vi "Write Valve.vi"(8 "error in (no error)":errorcluster, 11 "MFC in":refnum<class "Valve.lvclass">) -> (0 "error out":errorcluster, 3 "MFC out":refnum<class "Valve.lvclass">)   [LabVIEW 2013, in "Valve.lvlib" / "Valve.lvclass"]
uses:
  Valve.lvclass
  Valve.lvclass/Valve.ctl
  Read Valve Position.vi
  Read VISA.vi
  PluginInterface/PluginInterface.lvlibp/PluginInterfaceClass/Read DVR.vi
  PluginInterface/Actor Framework.lvlibp/Message Enqueuer/Enqueue.vi
  Valve Messages/Log Data Msg/Log Data Msg.lvclass
  Valve Messages/Update Graphs Msg/Update Graphs Msg.lvclass
  PluginInterface/Actor Framework.lvlibp/Actor/Actor.lvclass
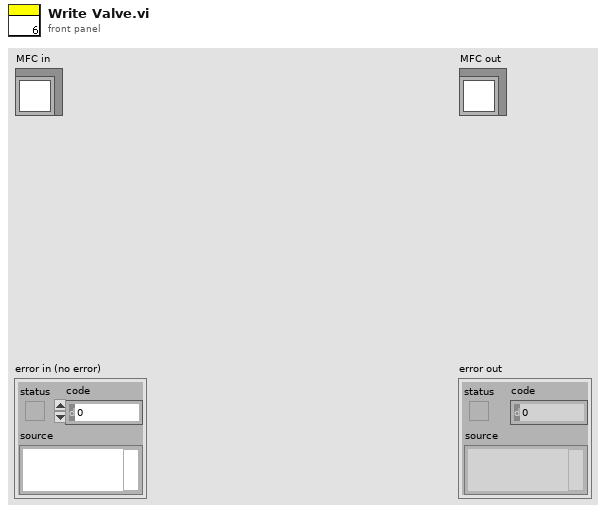
[diagram p1: front panel]
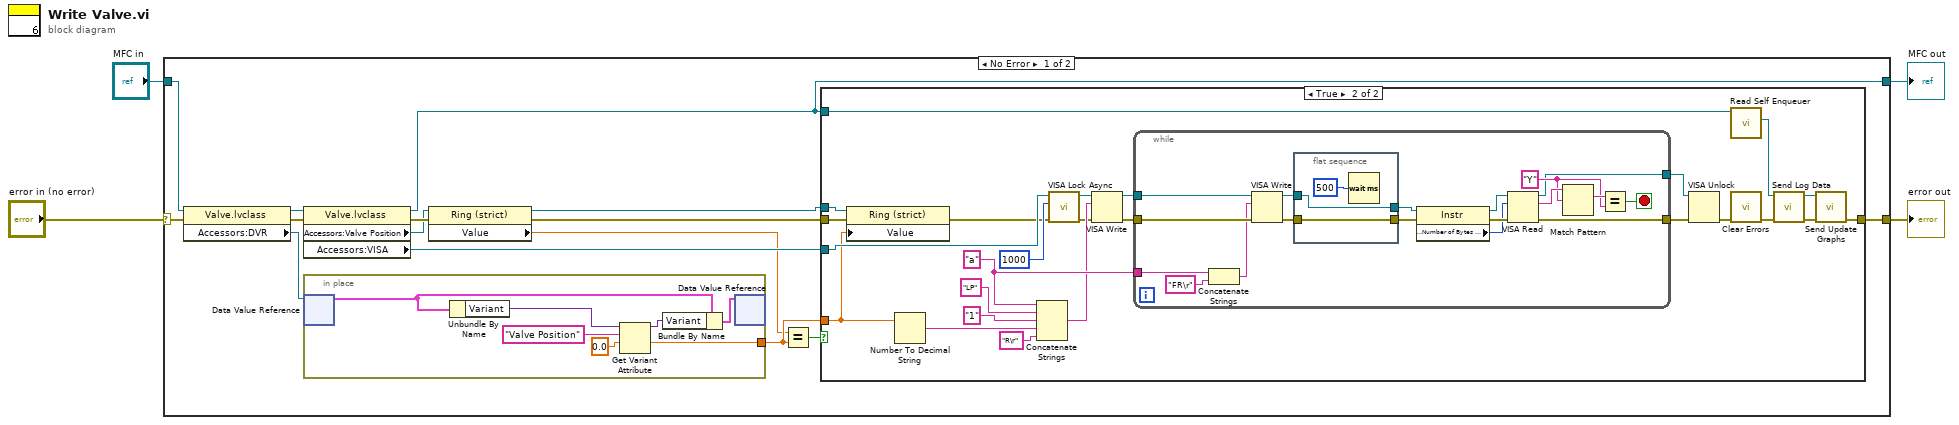
[diagram p0: block diagram]
diagram:
  n1 = case shown="No Error" "error in (no error)" {
    selector: "error in (no error)" -> [w18 w75]
    tunnel: [w12 w75] -> w1
    tunnel: [w5 w74] -> w2
    tunnel: "MFC in" -> [w19 w74]
    frame No Error {
      n2 = property class="Valve.lvclass"(reference=w19, error in=w18) -> (reference out=w17:refnum<class "Valve.lvclass">, error out=w15:errorcluster, "Accessors:DVR"=w16:refnum<data-value>)
      n3 = property class="Valve.lvclass"(reference=w17, error in=w15) -> (reference out=w5:refnum<class "Valve.lvclass">, error out=w14:errorcluster, "Accessors:Valve Position"=w13:refnum<vi>, "Accessors:VISA"=w11:refnum<visa-resource-name>)
      n4 = in-place {
        in-place-border: [w67] -> w7
        n5 = in-place-dvr #1(w16) -> (w70:cluster{"Array":string[], "Variant":variant})  [unwired: 1 out]
        n6 = Unbundle By Name(w70) -> ("Variant"=w72:variant)
        n7 = Get Variant Attribute(Variant=w72, name="Valve Position", default value (empty Variant)=0.0) -> (duplicate Variant=w71:variant, value=w67:dbl)  [unwired: 1 in, 2 out]
        n8 = Bundle By Name(cluster=w70, "Variant"=w71) -> (w73:cluster{"Array":string[], "Variant":variant})
        n9 = in-place-dvr #1(w73) -> ()  [unwired: 2 out]
      }
      n10 = property class="Ring (strict)"(reference=w13, error in=w14) -> (reference out=w10:refnum<vi>, error out=w9:errorcluster, "Value"=w6:dbl)
      n11 = Equal?(x=w6, y=w7) -> (x = y?=w8:bool)
      n12 = case shown="True" w8 {
        tunnel: [w20 w23] -> w12
        tunnel: w11 -> [_ w31]
        tunnel: w10 -> [_ w30]
        tunnel: w9 -> [w20 w29]
        tunnel: w7 -> [_ w27]
        tunnel: w5 -> [_ w22]
        frame False {
        }
        frame True {
          w45 = "a" ("String")
          n13 = property class="Ring (strict)"(reference=w30, error in=w29, "Value"=w27) -> (error out=w28:errorcluster)  [unwired: 1 out]
          n14 = Number To Decimal String(number=w27) -> (decimal integer string=w38:string)  [unwired: 1 in]
          n15 = Concatenate Strings(w45, "LP" ("string"), "1" ("string"), w38, "R\r" ("string")) -> (w40:string)
          n16 = call <vilib>:"VISA Lock Async.vi"("error in (no error)"=w28, "timeout (0)"=u32 1000, "VISA resource name"=w31) -> ("error out"=w34:errorcluster, "VISA resource name out"=w33:refnum<visa-resource-name>)  [unwired: 6 in, 1 out]
          n17 = VISA Write(VISA resource name=w33, write buffer=w40, error in (no error)=w34) -> (VISA resource name out=w43:refnum<visa-resource-name>, error out=w44:errorcluster)  [unwired: 1 out]
          n18 = while {
            tunnel: w43 -> [w56]
            tunnel: w44 -> [w55]
            tunnel: [w60] -> w37
            tunnel: w45 -> [w49]
            tunnel: [w47] -> w36
            stop <- w46 stop-if-true
            w57 = "Y" ("regular expression")
            n19 = Concatenate Strings(w49, "FR\r" ("write buffer")) -> (w48:string)
            n20 = VISA Write(VISA resource name=w56, write buffer=w48, error in (no error)=w55) -> (VISA resource name out=w54:refnum<visa-resource-name>, error out=w52:errorcluster)  [unwired: 1 out]
            n21 = flat-sequence {
              tunnel: [w65] -> w53
              tunnel: w54 -> [w65]
              tunnel: [w64] -> w51
              tunnel: w52 -> [w64]
              frame #0 {
                n22 = Wait (ms)(milliseconds to wait=u32 500) -> ()  [unwired: 1 out]
              }
            }
            n23 = property class="Instr"(reference=w53, error in=w51) -> (reference out=w63:refnum<visa-resource-name>, error out=w62:errorcluster, "Serial Settings:Number of Bytes at Serial Port"=w61:u32)
            n24 = VISA Read(VISA resource name=w63, byte count=w61, error in (no error)=w62) -> (VISA resource name out=w47:refnum<visa-resource-name>, read buffer=w59:string, error out=w60:errorcluster)  [unwired: 1 out]
            n25 = Match Pattern(string=w59, regular expression=w57) -> (match substring=w58:string)  [unwired: 1 in, 3 out]
            n26 = Equal?(x=w58, y=w57) -> (x = y?=w46:bool)
          }
          n27 = VISA Unlock(8:w37, 11:w36) -> (0:w35:errorcluster)  [unwired: 1 out]
          n28 = call "Read Self Enqueuer.vi"("Actor"=w22) -> ("Self Enqueuer"=w21:refnum<class "Message Enqueuer.lvclass">)  [unwired: 10 in]
          n29 = call <vilib>:"Clear Errors.vi"("error in (no error)"=w35) -> ("error out"=w25:errorcluster)  [unwired: 6 in]
          n30 = call "Send Log Data.vi"("error in (no error)"=w25, "Message Enqueuer"=w21) -> ("error out"=w24:errorcluster, "Message Enqueuer out"=w26:refnum<class "Message Enqueuer.lvclass">)  [unwired: 8 in]
          n31 = call "Send Update Graphs.vi"("error in (no error)"=w24, "Message Enqueuer"=w26) -> ("error out"=w23:errorcluster)  [unwired: 8 in, 1 out]
        }
      }
    }
    frame Error {
    }
  }
  "error out" <- w1
  "MFC out" <- w2
